vi "Close XML.vi"(8 "error in":errorcluster, 11 "StateValues":T1) -> (0 "error out":errorcluster)   [LabVIEW 2025]
uses:
  <vilib>/xml/NI_XML.lvlib
  <vilib>/xml/Close Reference(Node).vi
  Types/StateValues.ctl
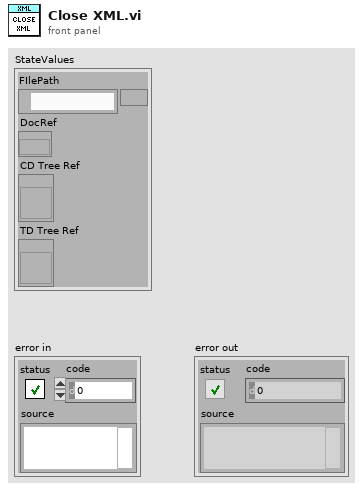
[diagram p1: front panel]
types:
  T1 = typedef "StateValues.ctl" = cluster{"FIlePath":path, "DocRef":refnum<k20>, "CD Tree Ref":refnum<vi>, "TD Tree Ref":refnum<vi>}
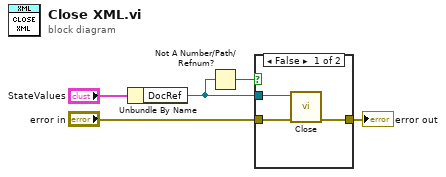
[diagram p0: block diagram]
diagram:
  n1 = Unbundle By Name("StateValues") -> ("DocRef"=w3:refnum<k20>)
  n2 = Not A Number/Path/Refnum?(number/path/refnum=w3) -> (NaN/Path/Refnum?=w4:bool)
  n3 = case shown="False" w4 {
    tunnel: w3 -> [w8 _]
    tunnel: [w7 w9] -> w2
    tunnel: "error in" -> [w6 w9]
    frame False {
      n4 = call-poly <vilib>:"Close.vi"("error in (no error)"=w6, "node"=w8) -> ("error out"=w7:errorcluster)  [unwired: 7 in]
    }
    frame True {
    }
  }
  "error out" <- w2
